vi "GetAlazar_SaveToFile.vi"(0 "AlazarCluster":T12, 1 "Digitizer Settings":T8={"Digitizer delay (us) "=0.0, "rf points per line"=2048, "lines per plane"=128, "Samp Rate (Hz)"=100000000.0, "Additional dig delay (us)"=0.0, "Voltage Scale"=0.4, "Pre-Looks"=0, "Offset delay (us)"=0.0, "bits A/D"=8, "Avg Num"=1, "DigTimeOut"=5.0, "Rel Dig Delay"=0.0, "Dig Ch"=0, "LeCroyCluster"={"LeCroy Channels"=[TRUE, FALSE, FALSE, FALSE], "LC read pt offset"=0.0, "Sweep Avg"=FALSE}, "Main Digitizer"=enum."NI Digitizer", "Dig Config"=enum."Single channel", "Digitizer ID Cluster"={"Acqiris/Alazar/SP ID"=[], "NI Instr Handles"=[], "LeCroy VISA"="", "GaGe Handle"={"Handle"=0, "Sample size"=0, "Resolution"=0, "Offset"=0, "Channels"=0, "Boards"=0}, "ATS Ref"="ATS9350", "Acqiris Address"=["PCI::INSTR0"], "ADQRef"=refnum, "adq_cu_ptr"=refnum}, "Trigger Settings"={"Trig Source"=1, "Trig Coupling"=0, "Trig Slope"=0, "Level (mV)"=1500.0}, "Bulk Acq"=FALSE, "Bulk Start Indexes"=[], "Data Ref RF"=refnum, "NI ID/Channel"=[], "Total Dig CH"=1, "Xtra Ann Trig delay (us)"=10.0, "Fix Z Delay?"=FALSE, "One Way Transmission?"=FALSE, "Data Ref Log"=refnum} {"Trigger Settings"."Trig Slope" items=["Positive", "Negative"]; "Trigger Settings"."Level (mV)" format="%.2f"; "Trigger Settings"."Trig Coupling" items=["DC 1 MOhm", "AC 1 MOhm", "DC 50 Ohm", "AC 50 Ohm"]; "Trigger Settings"."Trig Source" items=["Chan 1", "External"]; "Rel Dig Delay" format="%.2f"; "DigTimeOut" format="%.2f"; "Avg Num" min=1; "Offset delay (us)" format="%.2f"; "Additional dig delay (us)" format="%.2f"; "Digitizer delay (us)" format="%.2f"}, 4 "Ann Array Params":T1={"Synth Foc?"=FALSE, "Focal Zones"=41, "Switch T/R"=0, "Trans Geometry (mm)"={"Transducer"=0, "Geo Focus"=12.0, "a (radius)"=3.0, "# of rings"=5, "kerf space "=0.1, "Center Freq"=12.0}, "Sub Ap Excite?"=FALSE, "Full Array Scan?"=FALSE, "Xmt/Rcv"={"XMIT"=[TRUE, TRUE, TRUE, TRUE, TRUE], "RCV"=[TRUE, TRUE, TRUE, TRUE, TRUE]}, "PulseSpacing (us)"=0.0, "Xmit Ring"=0, "XMIT CHS"=0, "RCV CHS"=0, "GPU?"=FALSE, "Save TIFF?"=FALSE, "downfactor"=1, "RCV 1CH"=0} {"RCV 1CH" items=["All", "1", "2", "3", "4", "5"]; "Trans Geometry (mm)"."Transducer" items=["6D 12R 40 MHz"=0, "10D 31R 20 MHz"=1, "10D 23R 20 MHz"=2, "6D 23R 40 MHz"=3, "4.5D 10.7R 40 MHz"=4, "9D 23.5R 20 MHz"=5, "9D 25.8R 20MHz"=6, "Enter"=99]; "Switch T/R" min=1 max=5 step=1}, 7 "errorin":errorcluster, 8 "File Array":string[](array[string]), 9 "Motion Settings":T4={"No Motion?"=FALSE, "Motion System"=enum."NI 735x", "Motion Bd ID"=1, "Motion Profile"="SMAC1", "# Axis"=1, "Reverse Z axis?"=TRUE, "SMAC Axis"=0, "scan pair"=enum."y-(x) scan", "RT fps"=6.0, "Steps per mm"=[1000, 1000, 1000, 1000], "Motor Parameters"={"velocity ct/s"=[10000.0, 10000.0, 10000.0, 50000.0], "accel ct/s^2"=[50000.0, 50000.0, 50000.0, 200000.0]}, "One Way Scan"=FALSE, "Reverse One Way Scan"=FALSE, "Global Position (mm)"=[], "Plane"=0, "Distance between\nscan lines (um)"=0.0, "Distance between\nscan planes (um)"=0.0, "number of scan planes"=1, "Total steps in line"=0, "Xtra plane\ndistance  (um)"=100, "Xtra planes "=1, "Add Axis"=FALSE, "overshoot cts"=200, "BKPT Shift"=0, "Scan Start Time (ms)"=0, "ESP VISA"="GPIB::1::INSTR", "3rd Axis"=1, "GL Ref Out"=refnum, "Galil Address"=""} {"3rd Axis" items=["x", "y", "z", "w"]; "Xtra planes" min=1; "Xtra plane\ndistance  (um)" min=0; "Distance between\nscan planes (um)" format="%.2f"; "Distance between\nscan lines (um)" format="%.2f"; "SMAC Axis" items=["None"=0, "Axis 1"=1, "Axis 2"=2, "Axis 3"=3, "Axis 4"=4, "Axis 5"=5, "Axis 6"=6, "Axis 7"=7, "Axis 8"=8, "Vector Space 1"=17, "Vector Space 2"=18, "Vector Space 3"=19, "Vector Space 4"=20]; "Motion Bd ID" min=1 max=32 step=1}, 10 "lines per plane":i32, 15 "Reverse?":bool) -> (17 "Raw VGain (scale)":dbl, 18 "Gain Array":T14(array[cluster]), 21 "VGain (dB)":dbl, 27 "error out":errorcluster)   [LabVIEW 2022 SP3]
uses:
  -ScanSystem/DataHandling/ReverseData.vi
  -DigitizerRoutines/DigitizerSettings.ctl
  -DigitizerRoutines/DigitizerID.ctl
  -DigitizerRoutines/Digitizer.ctl
  Motion Controllers/NI_controller/-NI_MotionRoutines/MotionSys.ctl
  Motion Controllers/-MotionRoutines/ScanAxis.ctl
  Motion Controllers/NI_controller/-NI_MotionRoutines/MotionParameters.ctl
  Annular Array/-AnnularRoutines/ArrayGeometry.ctl
  Annular Array/-AnnularRoutines/TransGeometry.ctl
  Annular Array/-AnnularRoutines/AnnularArray.ctl
  -DigitizerRoutines/DigConfig.ctl
  Motion Controllers/-MotionRoutines/3rdAxis.ctl
  C:/Windows/System32/ADQAPI_dotNet_helper.dll
panel:
  out "Voltage Scale":T13
  # "1-D and 2-D B scan settings"
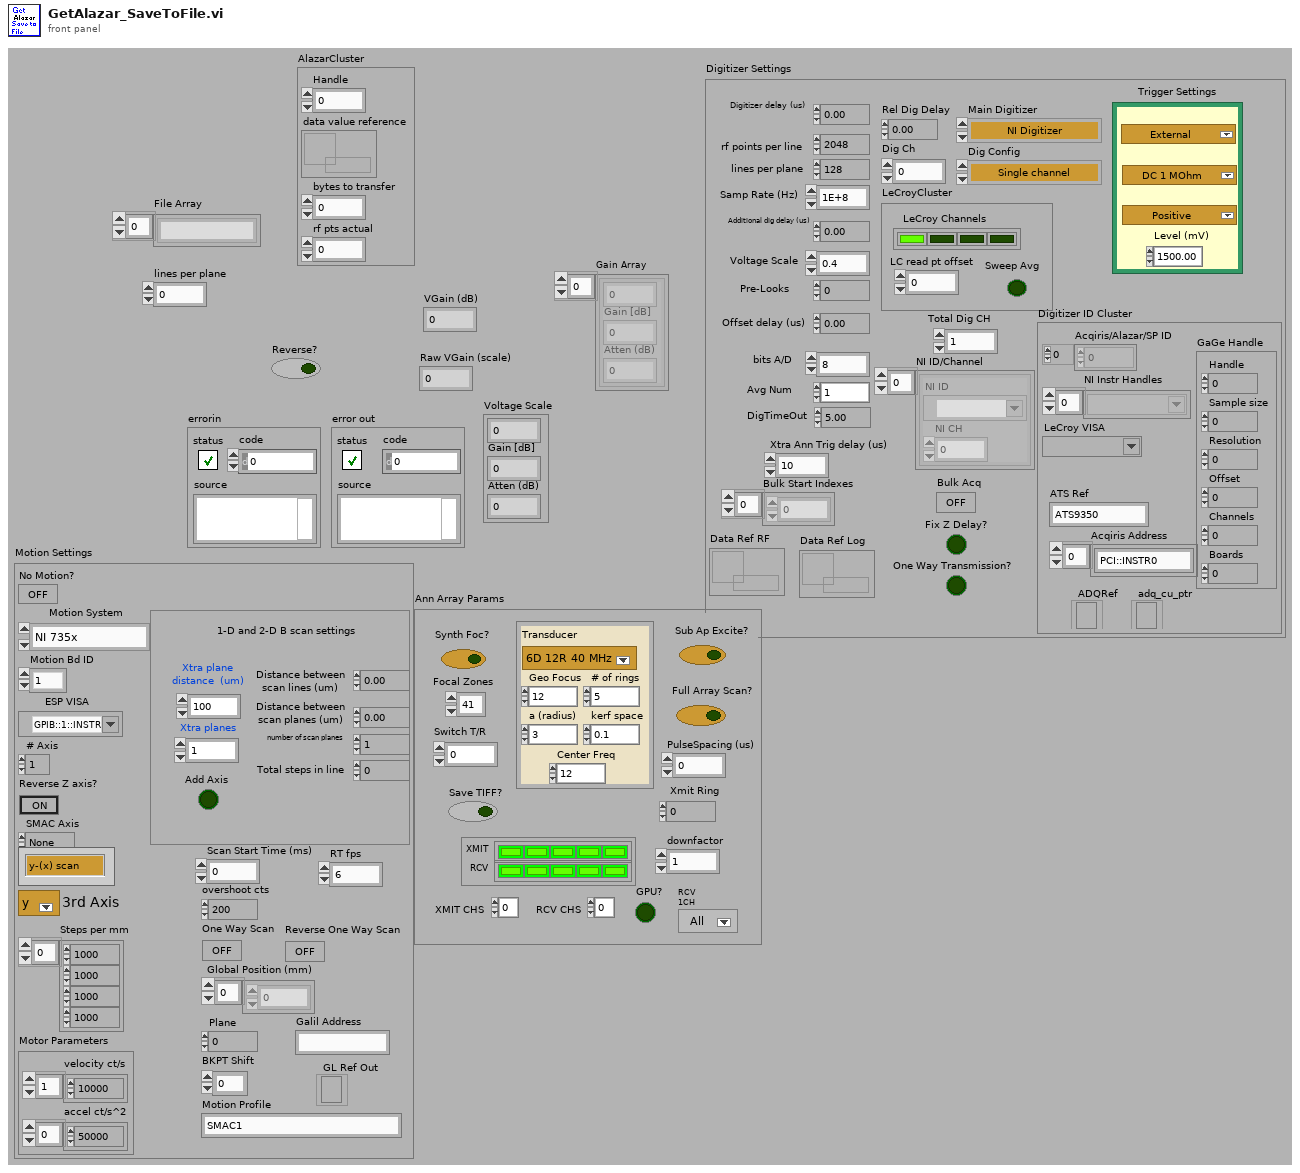
[diagram p1: front panel]
types:
  T1 = typedef "AnnularArray.ctl" = cluster{"Synth Foc?":bool, "Focal Zones":i16, "Switch T/R":i16, "Trans Geometry (mm)":T2, "Sub Ap Excite?":bool, "Full Array Scan?":bool, "Xmt/Rcv":cluster{"XMIT":bool[], "RCV":bool[]}, "PulseSpacing (us)":sgl, "Xmit Ring":i32, "XMIT CHS":u8, "RCV CHS":u8, "GPU?":bool, "Save TIFF?":bool, "downfactor":i32, "RCV 1CH":u16}
  T2 = typedef "TransGeometry.ctl" = cluster{"Transducer":T3, "Geo Focus":dbl, "a (radius)":dbl, "# of rings":i32, "kerf space ":dbl, "Center Freq":dbl}
  T3 = typedef "ArrayGeometry.ctl" = u16
  T4 = typedef "MotionParameters.ctl" = cluster{"No Motion?":bool, "Motion System":T5, "Motion Bd ID":u8, "Motion Profile":string, "# Axis":i8, "Reverse Z axis?":bool, "SMAC Axis":u16, "scan pair":T6, "RT fps":sgl, "Steps per mm":i32[], "Motor Parameters":cluster{"velocity ct/s":dbl[], "accel ct/s^2":dbl[]}, "One Way Scan":bool, "Reverse One Way Scan":bool, "Global Position (mm)":dbl[], "Plane":i32, "Distance between\nscan lines (um)":sgl, "Distance between\nscan planes (um)":sgl, "number of scan planes":i32, "Total steps in line":i32, "Xtra plane\ndistance  (um)":i32, "Xtra planes ":i32, "Add Axis":bool, "overshoot cts":i32, "BKPT Shift":i32, "Scan Start Time (ms)":u32, "ESP VISA":refnum<visa-resource-name>, "3rd Axis":T7, "GL Ref Out":refnum<k7>, "Galil Address":string}
  T5 = typedef "MotionSys.ctl" = enum16{"MM3000", "NI 735x", "Newport ESP", "No Motion Card", "Galil"}
  T6 = typedef "ScanAxis.ctl" = enum16{"y-(x) scan", "x-(y) scan", "z-(x) scan", "z-(y) scan", "y-(z) scan", "x-(z) scan", "w-(x) scan", "w-(y) scan", "w-(z) scan", "x-(w) scan", "y-(w) scan", "z-(w) scan"}
  T7 = typedef "3rdAxis.ctl" = u16
  T8 = typedef "DigitizerSettings.ctl" = cluster{"Digitizer delay (us) ":dbl, "rf points per line":i32, "lines per plane":i32, "Samp Rate (Hz)":dbl, "Additional dig delay (us)":dbl, "Voltage Scale":dbl, "Pre-Looks":i32, "Offset delay (us)":dbl, "bits A/D":i8, "Avg Num":i32, "DigTimeOut":sgl, "Rel Dig Delay":sgl, "Dig Ch":i32, "LeCroyCluster":cluster{"LeCroy Channels":bool[], "LC read pt offset":dbl, "Sweep Avg":bool}, "Main Digitizer":T9, "Dig Config":T10, "Digitizer ID Cluster":T11, "Trigger Settings":cluster{"Trig Source":u16, "Trig Coupling":u16, "Trig Slope":u16, "Level (mV)":dbl}, "Bulk Acq":bool, "Bulk Start Indexes":i32[], "Data Ref RF":refnum<data-value>, "NI ID/Channel":cluster{"NI ID":refnum<k15>, "NI CH":i32}[], "Total Dig CH":i32, "Xtra Ann Trig delay (us)":dbl, "Fix Z Delay?":bool, "One Way Transmission?":bool, "Data Ref Log":refnum<data-value>}
  T9 = typedef "Digitizer.ctl" = enum16{"Acqiris Digitizer", "NI Digitizer", "LeCroy", "GaGe", "AlazarTech", "No Digitizer", "Teledyne"}
  T10 = typedef "DigConfig.ctl" = enum16{"Single channel", "2 Chans w/ 2 Acqiris", "2 Chans w/ 1 Acqiris", "5-CH Pulser New", "5-CH pulser w/ ann array", "5-pass style ann array", "Empty"}
  T11 = typedef "DigitizerID.ctl" = cluster{"Acqiris/Alazar/SP ID":u32[], "NI Instr Handles":refnum<k15>[], "LeCroy VISA":refnum<visa-resource-name>, "GaGe Handle":cluster{"Handle":u32, "Sample size":u32, "Resolution":i32, "Offset":i32, "Channels":u32, "Boards":u32}, "ATS Ref":string, "Acqiris Address":string[], "ADQRef":refnum<k24>, "adq_cu_ptr":refnum<k24>}
  T12 = cluster{"Handle":u32, "data value reference":refnum<data-value>, "bytes to transfer":u32, "rf pts actual":u32}
  T13 = cluster{sgl, "Gain [dB]  ":sgl, "Atten (dB)":sgl}
  T14 = cluster{sgl, "Gain [dB]  ":sgl, "Atten (dB)":sgl}[]
  T15 = enum16{"big-endian, network order", "native, host order", "little-endian"}
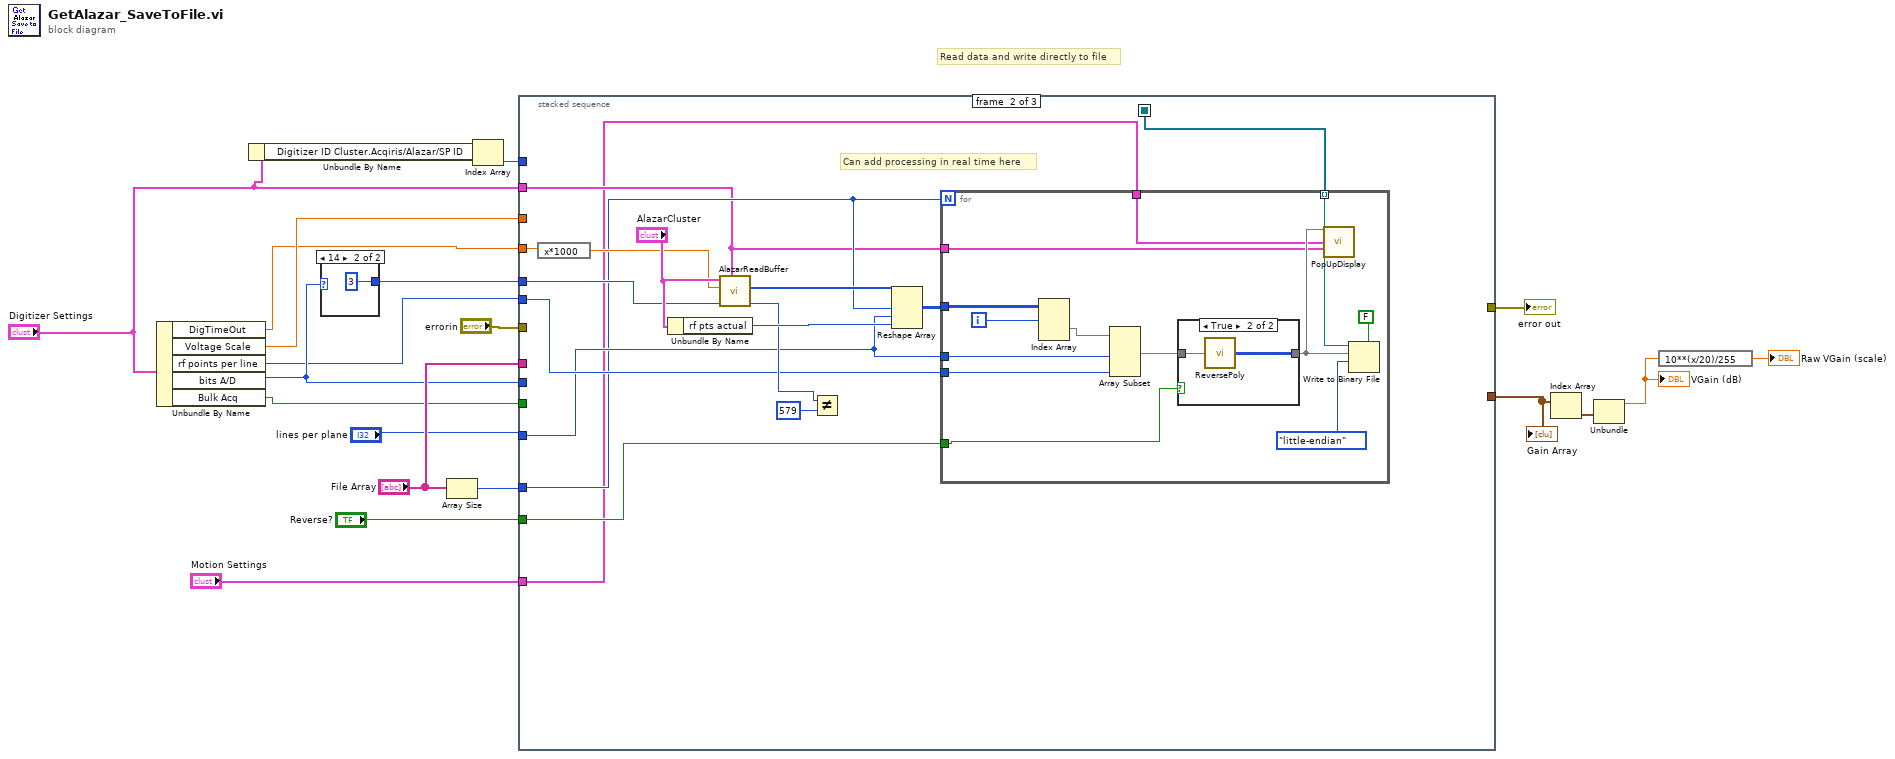
[diagram p0: block diagram]
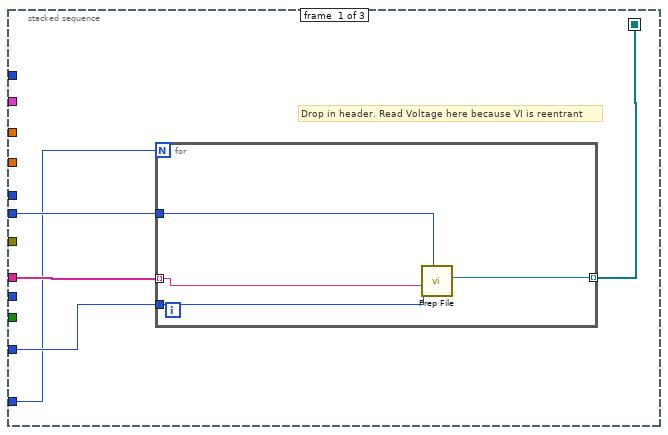
[diagram p3: hidden frame]
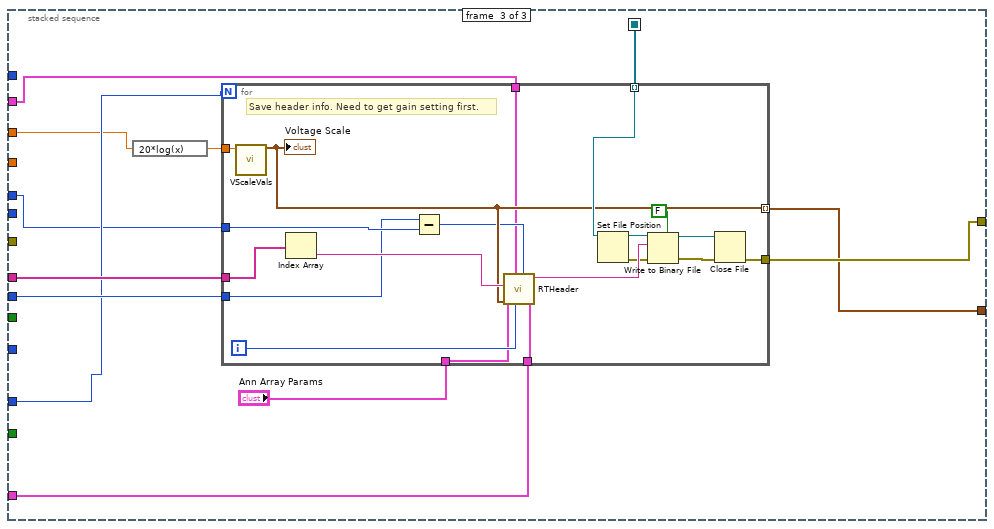
[diagram p5: hidden frame]
diagram:
  # "Read data and write directly to file"
  n1 = Unbundle By Name("Digitizer Settings") -> ("DigTimeOut"=w4:sgl, "Voltage Scale"=w5:dbl, "rf points per line"=w6:i32, "bits A/D"=w7:i8, "Bulk Acq"=w2:bool)
  n2 = Unbundle By Name("Digitizer Settings") -> ("Digitizer ID Cluster.Acqiris/Alazar/SP ID"=w10:u32[])
  n3 = case shown="14" w7 {
    tunnel: [_ u16 3 ("Extra Shift")] -> w8
    frame 0, Default {
    }
    frame 14 {
    }
  }
  n4 = Array Size(array="File Array") -> (size(s)=w17:i32)
  n5 = Index Array(array=w10) -> (element=w9:u32)  [unwired: 1 in]
  n6 = stacked-sequence {
    seq-local: [w26 _ _] -> [_ w37 w68]
    tunnel: [_ _ w74] -> w11
    tunnel: w4 -> [_ w36 _]
    tunnel: "lines per plane" -> [w23 w39 _]
    tunnel: w6 -> [w24 w40 _]
    tunnel: "File Array" -> [w25 _ w73]
    tunnel: "Reverse?" -> [_ w38 _]
    tunnel: "errorin" -> [_ _ _]
    tunnel: w17 -> [w22 w33 w69]
    tunnel: [_ _ w70] -> w13
    tunnel: w7 -> [_ _ w72]
    tunnel: w2 -> [_ _ _]
    tunnel: w9 -> [_ _ _]
    tunnel: w8 -> [_ w34 w67]
    tunnel: "Digitizer Settings" -> [_ w32 w65]
    tunnel: w5 -> [_ _ w66]
    tunnel: "Motion Settings" -> [_ w31 w63]
    frame #0 {
      # "Drop in header. Read Voltage here because VI is reentrant"
      n7 = for {
        N: w22 -> [_]
        tunnel: [w30] -> w26 mode=indexing
        tunnel: w25 -> [w27] mode=indexing
        tunnel: w24 -> [w29]
        tunnel: w23 -> [w28]
        n8 = call "Prep File.vi"("Num Samps"=w29, "Num Segs"=w28, "File Name"=w27) -> ("refnum out"=w30:refnum<file>)  [unwired: 4 in, 1 out]
      }
    }
    frame #1 {
      # "Can add processing in real time here"
      n9 = expression code="x*1000"(w36) -> (w35:sgl)
      n10 = Unbundle By Name("AlazarCluster") -> ("rf pts actual"=w44:u32)
      n11 = call "AlazarReadBuffer.vi"("Digitizer Settings"=w32, "Extra Shift"=w34, "time out"=w35, "AlazarCluster"="AlazarCluster") -> ("Return Code"=w43:u32, "Data Array"=w45:i16[])  [unwired: 5 in, 1 out]
      n12 = Not Equal?(x=w43, y=u32 579) -> ()  [unwired: 1 out]
      n13 = Reshape Array(w45, w33, w39, w44) -> (w46:i16[][][])
      n14 = for {
        N: w33 -> [_]
        tunnel: w46 -> [w59]
        tunnel: w40 -> [w58]
        tunnel: w39 -> [w57]
        tunnel: w38 -> [w56]
        tunnel: w37 -> [w52] mode=indexing
        tunnel: w32 -> [w48]
        tunnel: w31 -> [w47]
        i -> [w50]
        n15 = Index Array(array=w59, index (dim 0)=w50) -> (element=w51:i16[][])  [unwired: 2 in]
        n16 = Array Subset(array=w51, length (row)=w57, length (col)=w58) -> (w55:i16[][])  [unwired: 2 in]
        n17 = case shown="True" w56 {
          tunnel: [w60 w62] -> w49
          tunnel: w55 -> [w60 w61]
          frame False {
          }
          frame True {
            n18 = call-poly "ReversePoly.vi"("Array in"=w61) -> ("Array out"=w62:i16[][])
          }
        }
        n19 = call "PopUpDisplay.vi"("Data"=w49, "Motion Settings In"=w47, "Digitizer Settings"=w48) -> ()  [unwired: 13 in]
        n20 = Write to Binary File(file (use dialog)=w52, data=w49, 5:FALSE ("prepend array or string size? (T)"), 9:T15."little-endian" ("byte order (0:big-endian, network order)")) -> ()  [unwired: 2 in, 3 out]
      }
    }
    frame #2 {
      n21 = expression code="20*log(x)"(w66) -> (w71:dbl)
      n22 = for {
        N: w69 -> [_]
        tunnel: [w93] -> w74
        tunnel: w73 -> [w92]
        tunnel: w72 -> [w80]
        tunnel: [w82] -> w70 mode=indexing
        tunnel: w71 -> [w84]
        tunnel: w68 -> [w83] mode=indexing
        tunnel: w67 -> [w81]
        tunnel: w65 -> [w78]
        tunnel: w63 -> [w77]
        tunnel: "Ann Array Params" -> [w75]
        i -> [w76]
        # "Save header info. Need to get gain setting first."
        n23 = call "VScaleVals.vi"("Full Scale"=w84) -> ("Voltage Scale"=w82:T13)  [unwired: 8 in, 2 out]
        "Voltage Scale" <- w82
        n24 = Index Array(array=w92) -> (element=w85:string)  [unwired: 1 in]
        n25 = Subtract(x=w80, y=w81) -> (x-y=w79:u16)
        n26 = call "RTHeader.vi"("Motion Settings"=w77, "Dig Word Size"=w79, "Pulser Channel"=w76, "Digitizer Settings"=w78, "Votage scaling"=w82, "Ann Array Params"=w75, "File Name In"=w85) -> ("Header String Out"=w88:string)  [unwired: 3 in, 1 out]
        n27 = Set File Position(refnum=w83) -> (refnum out=w87:refnum<file>, error out=w86:errorcluster)  [unwired: 3 in]
        n28 = Write to Binary File(file (use dialog)=w87, data=w88, error in=w86, 5:FALSE ("prepend array or string size? (T)")) -> (refnum out=w90:refnum<file>, error out=w89:errorcluster)  [unwired: 2 in, 1 out]
        n29 = Close File(refnum=w90, error in=w89) -> (error out=w93:errorcluster)  [unwired: 1 out]
      }
    }
  }
  "Gain Array" <- w13
  "error out" <- w11
  n30 = Index Array(array=w13) -> (element=w18:T13)  [unwired: 1 in]
  n31 = Unbundle(w18) -> (w19:sgl)  [unwired: 2 out]
  "VGain (dB)" <- w19
  n32 = expression code="10**(x/20)/255"(w19) -> (→"Raw VGain (scale)":sgl)
